vi "MGI Write Anything.vi"(5 "Read/Write Options":T1={"TS Fmt"="%04Y%02m%02d %02H%02M%S%25u", "Int Fmt"="%d", "Delimiter"=""}, 7 "Format String (%#_13g)":string="%#_13g", 8 "Error In":errorcluster, 9 "Section Name (Name of \"Anything\")":string, 10 "Anything":variant, 11 "Path (dialog)":path) -> (0 "Error Out":errorcluster, 1 "Write Warnings":string, 2 "Section Replaced?":bool)   [LabVIEW 2024]
doc: "This VI is designed to write any data type to an INI file in human readable form. It will overwrite any data in the specified section of the INI file but leave other sections unchanged.\n\nAuthored by Robert C. Mortensen\nsupport@mooregoodideas.com\nwww.mooregoodideas.com\n\nCopyright (c) 2010, Moore Good Ideas, Inc.\n\nAll rights reserved.\n\nRedistribution and use in source and binary forms, with or without modification, are permitted provided that the following conditions are met:\n\n * Redistributions of source code must retain the above copyright notice, this list of conditions and the following disclaimer.\n * Redistributions in binary form must reproduce the above copyright notice, this list of conditions and the following disclaimer in the documentation and/or other materials provided with the distribution.\n * Neither the name of Moore Good Ideas, Inc. nor the names of its contributors may be used to endorse or promote products derived from this software without specific prior written permission.\n\nTHIS SOFTWARE IS PROVIDED BY THE COPYRIGHT HOLDERS AND CONTRIBUTORS \"AS IS\" AND ANY EXPRESS OR IMPLIED WARRANTIES, INCLUDING, BUT NOT LIMITED TO, THE IMPLIED WARRANTIES OF MERCHANTABILITY AND FITNESS FOR A PARTICULAR PURPOSE ARE DISCLAIMED. IN NO EVENT SHALL THE COPYRIGHT OWNER OR CONTRIBUTORS BE LIABLE FOR ANY DIRECT, INDIRECT, INCIDENTAL, SPECIAL, EXEMPLARY, OR CONSEQUENTIAL DAMAGES (INCLUDING, BUT NOT LIMITED TO, PROCUREMENT OF SUBSTITUTE GOODS OR SERVICES; LOSS OF USE, DATA, OR PROFITS; OR BUSINESS INTERRUPTION) HOWEVER CAUSED AND ON ANY THEORY OF LIABILITY, WHETHER IN CONTRACT, STRICT LIABILITY, OR TORT (INCLUDING NEGLIGENCE OR OTHERWISE) ARISING IN ANY WAY OUT OF THE USE OF THIS SOFTWARE, EVEN IF ADVISED OF THE POSSIBILITY OF SUCH DAMAGE."
uses:
  MGI RWA Options Cluster.ctl
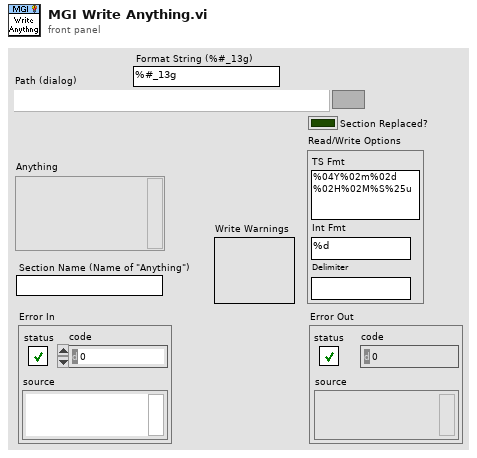
[diagram p1: front panel]
types:
  T1 = typedef "MGI RWA Options Cluster.ctl" = cluster{"TS Fmt":string, "Int Fmt":string, "Delimiter":string}
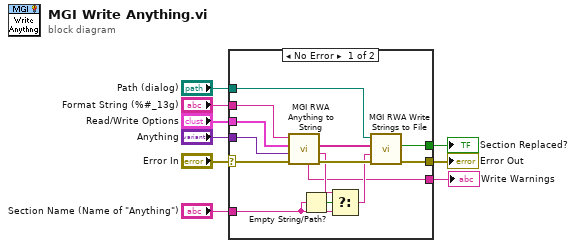
[diagram p0: block diagram]
diagram:
  n1 = case shown="No Error" "Error In" {
    selector: "Error In" -> [w10 w24]
    tunnel: "Anything" -> [w23 _]
    tunnel: [w22 w24] -> w8
    tunnel: "Path (dialog)" -> [w20 _]
    tunnel: "Format String (%#_13g)" -> [w19 _]
    tunnel: "Section Name (Name of \"Anything\")" -> [w16 _]
    tunnel: "Read/Write Options" -> [w14 _]
    tunnel: [w12 _] -> w3
    tunnel: [w11 _] -> w2
    frame No Error {
      n2 = call "MGI RWA Anything to String.vi"("Error In"=w10, "Anything"=w23, "Read/Write Options"=w14, "Format String (%#_13g)"=w19) -> ("Error Out"=w21:errorcluster, "Section"=w17:string, "Strings[]"=w13:string[], "Warnings"=w11:string)  [unwired: 4 in]
      n3 = Empty String/Path?(string/path=w16) -> (empty?=w18:bool)
      n4 = Select(t=w17, s=w18, f=w16) -> (s? t:f=w15:string)
      n5 = call "MGI RWA Write Strings to File.vi"("Error In"=w21, "Section Name"=w15, "Strings[]"=w13, "Path"=w20) -> ("Error Out"=w22:errorcluster, "Section Replaced?"=w12:bool)  [unwired: 6 in]
    }
    frame Error {
    }
  }
  "Error Out" <- w8
  "Section Replaced?" <- w3
  "Write Warnings" <- w2
